vi "MecaDrivePoseEst2_Execute.vi"(0 "Vision TImeStamp_Seconds":dbl=0.02, 3 "MecaPoseEst2Config":T2={"Rear Left Wheel M"={"X"=0.0, "Y"=0.0}, "Odom X std dev M"=0.02, "Odom Y std dev M"=0.02, "Odom Heading std dev Rad"=0.01, "Vision X std dev M"=0.1, "Vision Y std dev M"=0.1, "Vision Heading std dev Rad"=0.05, "Front Left Wheel M"={"X"=0.0, "Y"=0.0}, "Front Right Wheel M"={"X"=0.0, "Y"=0.0}, "Rear Right Wheel M"={"X"=0.0, "Y"=0.0}} {"Rear Right Wheel M"."Y" format="%14.3f"; "Rear Right Wheel M"."X" format="%14.3f"; "Front Right Wheel M"."Y" format="%14.3f"; "Front Right Wheel M"."X" format="%14.3f"; "Front Left Wheel M"."Y" format="%14.3f"; "Front Left Wheel M"."X" format="%14.3f"; "Vision Heading std dev Rad" format="%#_13g"; "Vision Y std dev M" format="%#_13g"; "Vision X std dev M" format="%#_13g"; "Odom Heading std dev Rad" format="%#_13g"; "Odom Y std dev M" format="%#_13g"; "Odom X std dev M" format="%#_13g"; "Rear Left Wheel M"."Y" format="%14.3f"; "Rear Left Wheel M"."X" format="%14.3f"}, 4 "visionRobotPose":T4={"TRANSLATION"={"X"=0.0, "Y"=0.0}, "ROTATION"={"VALUE"=0.0, "COS"=1.0, "SIN"=0.0}} {"ROTATION"."SIN" format="%13.4f"; "ROTATION"."COS" format="%13.4f"; "ROTATION"."VALUE" format="%13.4f"; "TRANSLATION"."Y" format="%14.3f"; "TRANSLATION"."X" format="%14.3f"}, 5 "Game Started":bool, 6 "Add Vision Meas":bool, 7 "InitialPose":T4={"TRANSLATION"={"X"=0.0, "Y"=0.0}, "ROTATION"={"VALUE"=0.0, "COS"=1.0, "SIN"=0.0}} {"ROTATION"."SIN" format="%13.4f"; "ROTATION"."COS" format="%13.4f"; "ROTATION"."VALUE" format="%13.4f"; "TRANSLATION"."Y" format="%14.3f"; "TRANSLATION"."X" format="%14.3f"}, 8 "Pass Through Time":dbl=-1.0, 9 "Gyro Degrees":dbl, 11 "Wheel Distances":T1 {"RearRight" format="%19.3f"; "RearLeft" format="%19.3f"; "FrontRight" format="%19.3f"; "FrontLeft" format="%19.3f"}) -> (1 "Error":bool, 2 "Estimated Pose":T4={"TRANSLATION"={"X"=0.0, "Y"=0.0}, "ROTATION"={"VALUE"=0.0, "COS"=1.0, "SIN"=0.0}} {"ROTATION"."SIN" format="%13.4f"; "ROTATION"."COS" format="%13.4f"; "ROTATION"."VALUE" format="%13.4f"; "TRANSLATION"."Y" format="%14.3f"; "TRANSLATION"."X" format="%14.3f"})   [LabVIEW 2019, in "Trajectory_Library.lvlib"]
uses:
  TypeDef/POSE2D.ctl
  TypeDef/TRANSLATION2D.ctl
  TypeDef/ROTATION2D.ctl
  Conv_Deg_Radians.vi
  Rotation2d_CreateAngle.vi
  Util_GetTime_U32.vi
  MatBuilder_Create.vi
  Util_GetTime_U64.vi
  Trajectory_Library.lvlib
  TypeDef/MECA_WHEEL_POSITIONS.ctl
  TypeDef/MECA_DRIVE_POSE_EST2_CONFIG.ctl
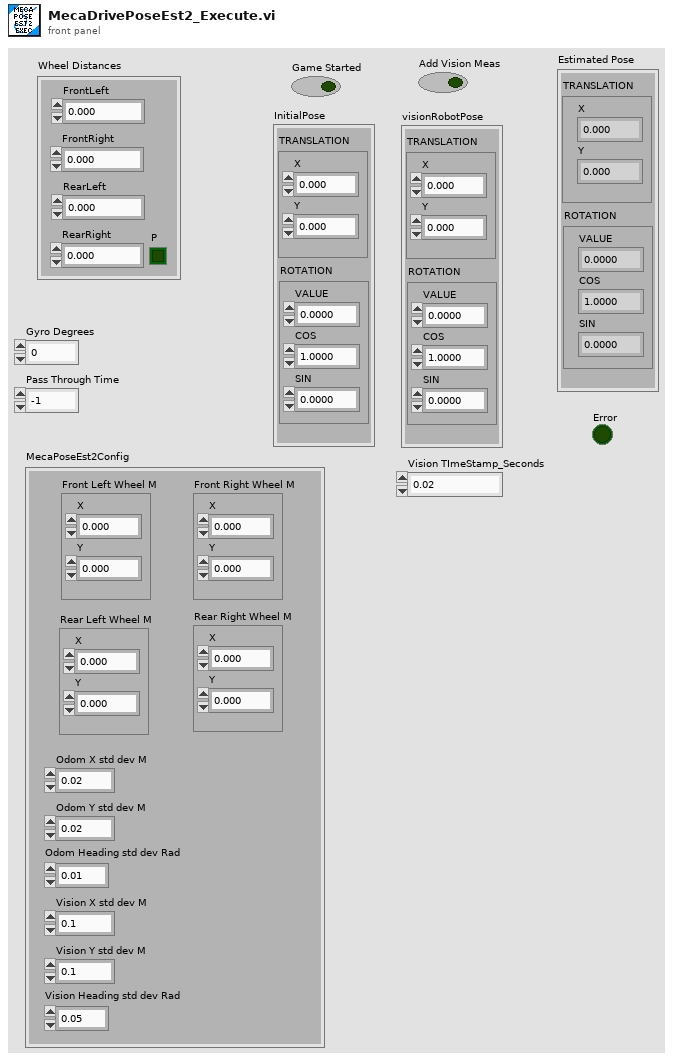
[diagram p1: front panel]
types:
  T1 = typedef "Trajectory_Library.lvlib/MECA_WHEEL_POSITIONS.ctl" = cluster{"FrontLeft":dbl, "FrontRight":dbl, "RearLeft":dbl, "RearRight":dbl, "P":bool}
  T2 = typedef "Trajectory_Library.lvlib/MECA_DRIVE_POSE_EST2_CONFIG.ctl" = cluster{"Rear Left Wheel M":T3, "Odom X std dev M":dbl, "Odom Y std dev M":dbl, "Odom Heading std dev Rad":dbl, "Vision X std dev M":dbl, "Vision Y std dev M":dbl, "Vision Heading std dev Rad":dbl, "Front Left Wheel M":T3, "Front Right Wheel M":T3, "Rear Right Wheel M":T3}
  T3 = typedef "Trajectory_Library.lvlib/TRANSLATION2D.ctl" = cluster{"X":dbl, "Y":dbl}
  T4 = typedef "Trajectory_Library.lvlib/POSE2D.ctl" = cluster{"TRANSLATION":T3, "ROTATION":T5}
  T5 = typedef "Trajectory_Library.lvlib/ROTATION2D.ctl" = cluster{"VALUE":dbl, "COS":dbl, "SIN":dbl}
  T6 = typedef "NI_Matrix.lvlib/RealMatrix.ctl" = dbl[][]
  T7 = typedef "Trajectory_Library.lvlib/MECA_DRIVE_KINEMATICS.ctl" = cluster{"FrontLeft":T3, "FrontRight":T3, "RearLeft":T3, "RearRight":T3, "InverseKinematics":T6, "ForwardKinematics":T6, "PrevCoR":T3}
  T8 = typedef "Trajectory_Library.lvlib/MECA_DRIVE_POSE_EST2.ctl" = cluster{"M_Vision_K":T6, "m_nominal_dT":dbl, "m_PrevTime_Sec":dbl, "Pose_Buffer":T9, "Meca_Drive_Odom":T10, "M_Q":T6}
  T9 = typedef "Trajectory_Library.lvlib/TIME_INTERPOLATABLE_VARIANT.ctl" = cluster{"TimeStamps":dbl[], "DataArray":variant[], "Min_TimeStamp":dbl, "Max_TimeStamp":dbl, "ItemCount":i32, "MaxBufferTime":dbl}
  T10 = typedef "Trajectory_Library.lvlib/MECA_DRIVE_ODOMETRY.ctl" = cluster{"POSE":T4, "GyroOffset":T5, "PreviousAngle":T5, "Kinematics":T7, "PreviousWheelPositions":T1}
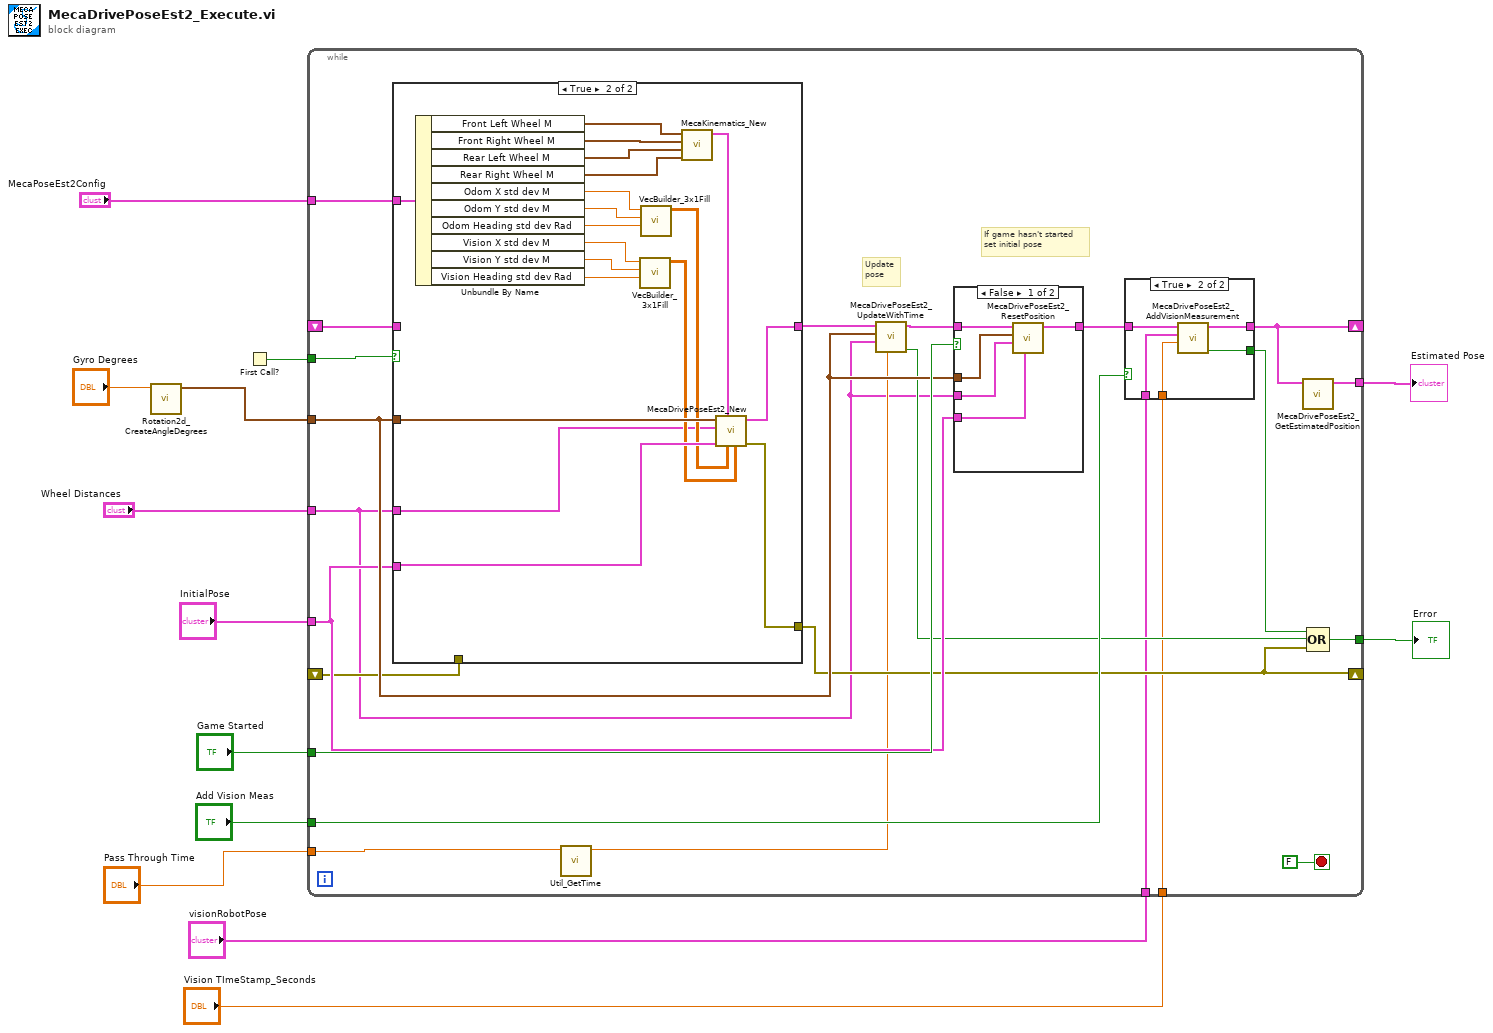
[diagram p0: block diagram]
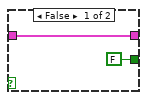
[diagram p3: hidden frame]
diagram:
  n1 = call "Rotation2d_CreateAngleDegrees.vi"("Angle_Degrees"="Gyro Degrees") -> ("ROTATION"=w4:T5)  [unwired: 10 in]
  n2 = First Call?() -> (First Call?: T/F=w13:bool)
  n3 = while {
    tunnel: w13 -> [w35]
    tunnel: w4 -> [w31]
    tunnel: "InitialPose" -> [w30]
    tunnel: "Game Started" -> [w32]
    shift-right: [w23] -> _
    shift-left: _ -> [w28]
    tunnel: "Add Vision Meas" -> [w27]
    shift-right: [w24] -> _
    shift-left: _ -> [w18]
    tunnel: [w22] -> w9
    tunnel: [w21] -> w8
    tunnel: "visionRobotPose" -> [w20]
    tunnel: "Vision TImeStamp_Seconds" -> [w19]
    tunnel: "Pass Through Time" -> [w16]
    tunnel: "MecaPoseEst2Config" -> [w15]
    tunnel: "Wheel Distances" -> [w14]
    stop <- FALSE stop-if-true
    # "If game hasn't started\nset initial pose"
    # "Update\npose"
    n4 = case shown="True" w35 {
      tunnel: w31 -> [_ w70]
      tunnel: w30 -> [_ w69]
      tunnel: [w50 w68] -> w24
      tunnel: [w51 w67] -> w34
      tunnel: w28 -> [w51 _]
      tunnel: w18 -> [w50 _]
      tunnel: w15 -> [_ w66]
      tunnel: w14 -> [_ w57]
      frame False {
      }
      frame True {
        n5 = Unbundle By Name(w66) -> ("Front Left Wheel M"=w55:T3, "Front Right Wheel M"=w54:T3, "Rear Left Wheel M"=w53:T3, "Rear Right Wheel M"=w52:T3, "Odom X std dev M"=w65:dbl, "Odom Y std dev M"=w64:dbl, "Odom Heading std dev Rad"=w63:dbl, "Vision X std dev M"=w62:dbl, "Vision Y std dev M"=w61:dbl, "Vision Heading std dev Rad"=w60:dbl)
        n6 = call "VecBuilder_3x1Fill.vi"("R2"=w60, "R1"=w61, "R0"=w62) -> ("output matrix"=w58:T6)  [unwired: 8 in]
        n7 = call "VecBuilder_3x1Fill.vi"("R2"=w63, "R1"=w64, "R0"=w65) -> ("output matrix"=w59:T6)  [unwired: 8 in]
        n8 = call "MecaKinematics_New.vi"("RearRight"=w52, "RearLeft"=w53, "FrontRight"=w54, "FrontLeft"=w55) -> ("MECA_DRIVE_KINEMATICS"=w56:T7)  [unwired: 7 in]
        n9 = call "MecaDrivePoseEst2_New.vi"("VisionMeasurementStdDevs"=w58, "StateStdDevs"=w59, "MECA_DRIVE_KINEMATICS"=w56, "InitialPose"=w69, "Module Positions"=w57, "gyroAngle"=w70) -> ("Error"=w68:errorcluster, "MecaDrivePoseEstimate"=w67:T8)  [unwired: 4 in]
      }
    }
    n10 = call "Util_GetTime.vi"("Pass_Through_Time"=w16) -> ("FPGA_Time_Seconds"=w17:dbl)  [unwired: 8 in, 2 out]
    n11 = call "MecaDrivePoseEst2_UpdateWithTime.vi"("CurrentTimeSeconds"=w17, "module Positions"=w14, "GyroAngle"=w31, "in MecaDrivePoseEst2"=w34) -> ("Error"=w26:bool, "Out MecaDrivePoseEst2"=w33:T8)  [unwired: 5 in, 1 out]
    n12 = case shown="False" w32 {
      tunnel: w33 -> [w41 w42]
      tunnel: w31 -> [w40 _]
      tunnel: w14 -> [w39 _]
      tunnel: w30 -> [w38 _]
      tunnel: [w37 w42] -> w29
      frame False {
        n13 = call "MecaDrivePoseEst2_ResetPosition.vi"("Pose"=w38, "Module Positions"=w39, "Gyro"=w40, "in MecaDrivePoseEst2"=w41) -> ("Out MecaDrivePoseEst2"=w37:T8)  [unwired: 7 in]
      }
      frame True {
      }
    }
    n14 = case shown="True" w27 {
      tunnel: w29 -> [w44 w49]
      tunnel: [w44 w48] -> w23
      tunnel: [FALSE ("Error") w47] -> w25
      tunnel: w20 -> [_ w46]
      tunnel: w19 -> [_ w45]
      frame False {
      }
      frame True {
        n15 = call "MecaDrivePoseEst2_AddVisionMeasurement.vi"("TImeStamp_Seconds"=w45, "visionRobotPose"=w46, "in MecaDrivePoseEst2"=w49) -> ("Error"=w47:bool, "Out MecaDrivePoseEst2"=w48:T8)  [unwired: 7 in]
      }
    }
    n16 = call "MecaDrivePoseEst2_GetEstimatedPosition.vi"("in MecaDrivePoseEstimate"=w23) -> ("Estimated Pose"=w22:T4)  [unwired: 10 in]
    n17 = Compound Arithmetic op=OR(w25, w26, w24) -> (w21:bool)
  }
  "Estimated Pose" <- w9
  "Error" <- w8
